vi "Open_Instr.vi"(8 "error in (no error)":errorcluster caption="entrée d'erreur (pas d'erreur)", 11 "Class Firebase Altyor en entrée":refnum<class "Class Instrument Database Altyor.lvclass">) -> (0 "error out":errorcluster caption="sortie d'erreur", 3 "Class  Firebase Altyor en sortie":refnum<class "Class Instrument Database Altyor.lvclass">)   [LabVIEW 2020, in "Library Instrument & Equipement.lvlib" / "Library Instruments.lvlib" / "Class Instrument Database Altyor.lvclass"]
uses:
  Class Instrument Database Altyor.lvclass
  Class Instrument Database Altyor.lvclass/Class Instrument Database Altyor.ctl
  Database/Database Altyor/Database Altyor.lvclass
  C:/Users/ngarcin/OneDrive - Altyor/Standard TB/Class/Database/Database drivers/Database Drivers.lvclass
  Instrument (Default)/Class Instrument (Default).lvclass
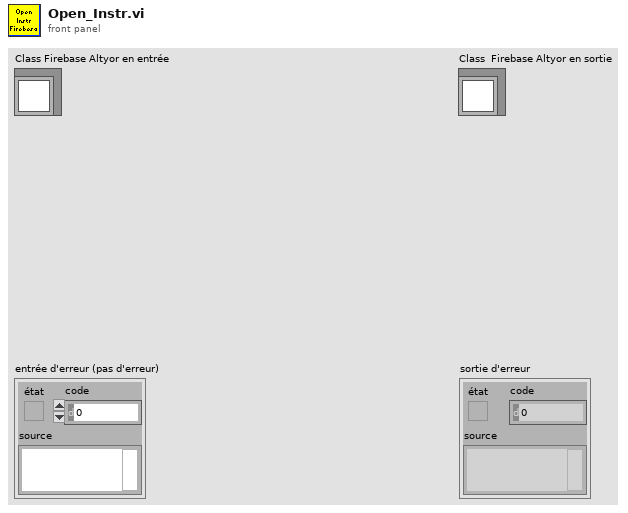
[diagram p1: front panel]
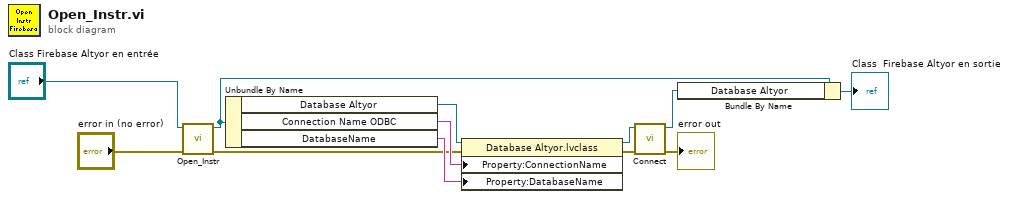
[diagram p0: block diagram]
diagram:
  n1 = call-parent "Open_Instr.vi"("error in (no error)"="error in (no error)", "Class Multimeter (Default) en entrée"="Class Firebase Altyor en entrée") -> ("error out"=w5:errorcluster, "Class Multimeter (Default) en sortie"=w10:refnum<class "Class Instrument Database Altyor.lvclass">)  [unwired: 8 in]
  n2 = Unbundle By Name(w10) -> ("Database Altyor"=w6:refnum<class "Database Altyor.lvclass">, "Connection Name ODBC"=w12:string, "DatabaseName"=w11:string)
  n3 = property class="Database Altyor.lvclass"(reference=w6, error in=w5, "Property:ConnectionName"=w12, "Property:DatabaseName"=w11) -> (reference out=w1:refnum<class "Database Altyor.lvclass">, error out=w4:errorcluster)
  n4 = call-dynamic "Connect.vi"("error in (no error)"=w4, "Database Altyor en entrée"=w1) -> ("error out"=→"error out":errorcluster, "Database Altyor en sortie"=w2:refnum<class "Database Altyor.lvclass">)  [unwired: 8 in]
  n5 = Bundle By Name(cluster=w10, "Database Altyor"=w2) -> (→"Class  Firebase Altyor en sortie":refnum<class "Class Instrument Database Altyor.lvclass">)
